vi "Stimulus-Set Level (array).vi"(0 "AO Control in":T1[](array[typedef]) {"Filter"."IIR Filter Cluster"."Forward Coefficients" format="%.4f"; "Filter"."IIR Filter Cluster"."Reverse Coefficients" format="%.4f"}, 1 "Apply multiplier? (F)":bool, 5 "Waveform in":dbl[][](array[numeric]), 11 "error in (no error)":errorcluster) -> (4 "AO Control out":T23(array[cluster]) {"Filter"."IIR Filter Cluster"."Forward Coefficients" format="%.4f"; "Filter"."IIR Filter Cluster"."Reverse Coefficients" format="%.4f"}, 6 "Waveform out":dbl[][](array[numeric]), 8 "Multipliers":dbl[](array[numeric]), 10 "Gains":dbl[](array[numeric]), 14 "Ceilings":dbl[](array[numeric]), 15 "error out":errorcluster)   [LabVIEW 2020]
uses:
  Controls/Waveform XCtl/Waveform Data.ctl
  Controls/Waveform XCtl/Waveform Enum.ctl
  Waveform VIs/Tone VIs/Tone Params.ctl
  Waveform VIs/Pulse Train VIs/Pulse Train Params.ctl
  Waveform VIs/Pulse Train VIs/Pulse Polarity.ctl
  Waveform VIs/Pulse Train VIs/PT-Continuous State.ctl
  Waveform VIs/Noise VIs/Noise Params.ctl
  Waveform VIs/File VIs/StimFile-Params.ctl
  Waveform VIs/FM Sweep VIs/FM Sweep Params.ctl
  Waveform VIs/Chirp Train VIs/Chirp Train.ctl
  Waveform VIs/Chirp Train VIs/Chirp Train Params.ctl
  Waveform VIs/Complex Tone VIs/CT-Params.ctl
  Waveform VIs/Complex Tone VIs/CT-Phase Enum.ctl
  Waveform VIs/Complex Tone VIs/CT-Runtime Data.ctl
  Waveform VIs/Moving Ripple VIs/Moving Ripple.ctl
  Waveform VIs/Moving Ripple VIs/Moving Ripple.Params.ctl
  Waveform VIs/Moving Ripple VIs/Moving Ripple.Data.ctl
  Controls/Filter XCtl/Filter Data.ctl
  Controls/Gate XCtl/Gate Data.ctl
  Controls/Level XCtl/Level Data.ctl
  Controls/Level XCtl/Level Units.ctl
  Controls/Stimulus Channel XCtl/Stimulus Channel Data.ctl
  PXI DAQ VIs/DAQ Engine VIs/AO Gain and Multiplier VIs/PXI Multipliers to AO Gains (1D).vi
  Controls/Waveform XCtl/Waveform XCtl.xctl
  Controls/Filter XCtl/Filter XCtl.xctl
  Controls/Gate XCtl/Gate Control.xctl
  Controls/Level XCtl/Level XCtl.xctl
  Controls/Stimulus Channel XCtl/Stimulus Channel.xctl
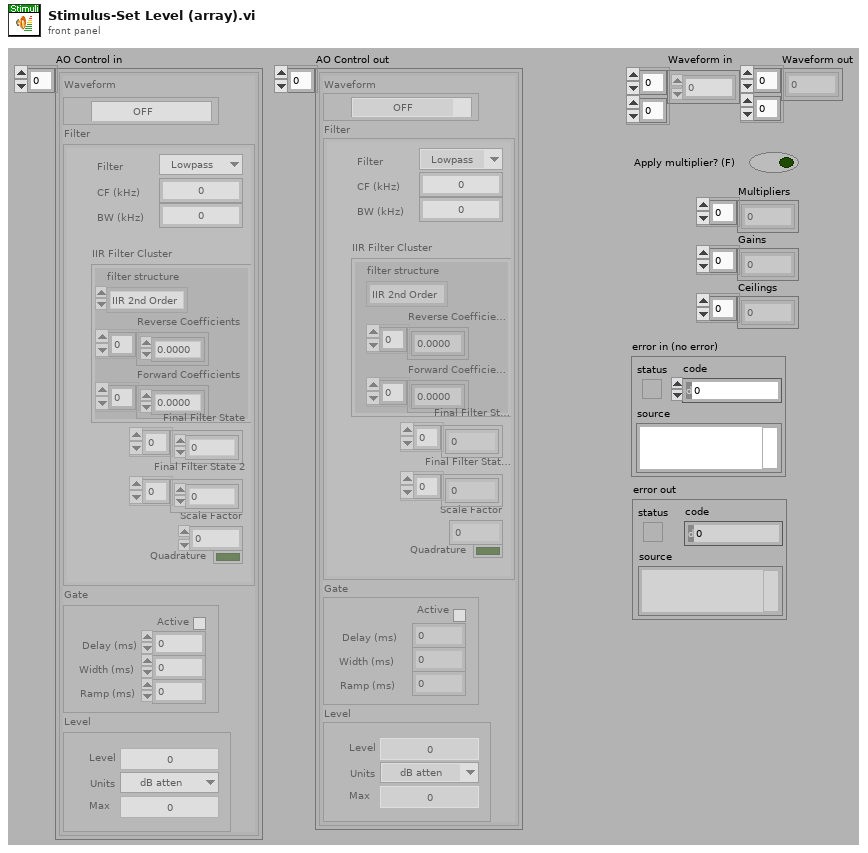
[diagram p1: front panel]
types:
  T1 = typedef "Stimulus Channel.xctl/Stimulus Channel Data.ctl" = cluster{"Waveform":T2, "Filter":T19, "Gate":T20, "Level":T21}
  T2 = typedef "Waveform XCtl.xctl/Waveform Data.ctl" = cluster{"Type":T3, "Tone":T4, "Pulse Train":T5, "Noise":T8, "File":T9, "FMSweep":T10, "Chirp Train":T11, "Complex Tone":cluster{"Params":T13, "Data":T15}, "Moving Ripple":T16}
  T3 = typedef "Waveform Enum.ctl" = enum16{"OFF", "Tone", "Noise", "Pulse Train", "File", "FM Sweep", "Chirp Train", "Complex Tone", "FM Tone", "Moving Ripple"}
  T4 = typedef "Tone Params.ctl" = cluster{"Frequency (kHz)":dbl, "Last Freq":dbl, "Last Phase":dbl}
  T5 = typedef "Pulse Train Params.ctl" = cluster{"Pulse width (us)":dbl, "Pulse rate (Hz)":dbl, "Gap (ms)":dbl, "Polarity":T6, "PT State":T7, "Asynch":bool}
  T6 = typedef "Pulse Polarity.ctl" = enum16{"POS", "NEG", "POS-NEG", "NEG-POS"}
  T7 = typedef "PT-Continuous State.ctl" = cluster{"Template":dbl[], "Nperiod":i32, "Index":i32, "Pulse Rate (Hz)":dbl, "Phase (cycles)":dbl, "Noff":i32}
  T8 = typedef "Noise Params.ctl" = cluster{"InvFilt":bool, "Noise":dbl[], "CurPt":i32, "Aweight":bool, "Seed":i32, "afile":path}
  T9 = typedef "StimFile-Params.ctl" = cluster{"Filename":path, "Signal":dbl[], "Channel":i32, "stream":bool, "offset":i32, "nreps":i32, "loops":i32, "Randomize":bool, "order":i32[], "Seed":i32, "Tokens":i32}
  T10 = typedef "FM Sweep Params.ctl" = cluster{"Rate (oct/s)":dbl, "Fmin (Hz)":dbl, "Fmax (Hz)":dbl, "Ramp (ms)":dbl, "Linear":bool}
  T11 = typedef "Chirp Train.ctl" = cluster{"Params":T12, "Data":cluster{"WF":dbl[]}}
  T12 = typedef "Chirp Train Params.ctl" = cluster{"Fmin (kHz)":dbl, "Fmax (kHz)":dbl, "Compensate":bool, "Duration (ms)":dbl}
  T13 = typedef "CT-Params.ctl" = cluster{"F0 (Hz)":dbl, "Band":cluster{"Flow (Hz)":dbl, "Fhigh (Hz)":dbl}, "Phase":T14, "Min F0 (Hz)":dbl, "Max F0 (Hz)":dbl, "ContinRandPhase":bool, "Max peak factor":dbl, "Max mod depth":dbl, "MinHarmNum":i32, "MaxHarmNum":i32, "Level Mode":enum16{"per component", "overall rms"}, "% jitter":dbl}
  T14 = typedef "CT-Phase Enum.ctl" = enum16{"Cosine", "Random", "Alternating"}
  T15 = typedef "CT-Runtime Data.ctl" = cluster{"Ncomp":i32, "MinHarm":i32, "Phase":dbl[], "Amplitude":dbl[], "Npts/frame":i32, "Last F0":dbl, "Fmin":dbl, "Fmax":dbl, "Lslope":dbl, "randphase":bool, "overall rms":bool, "fmult":dbl[], "jittered":bool}
  T16 = typedef "Moving Ripple.ctl" = cluster{"Params":T17, "Data":T18}
  T17 = typedef "Moving Ripple.Params.ctl" = cluster{"Fmin":dbl, "Fmax":dbl, "Density":dbl, "Velocity":dbl, "Depth":dbl, "Phase":dbl, "Comp/oct":i32}
  T18 = typedef "Moving Ripple.Data.ctl" = cluster{"Freq":dbl[], "A":dbl[], "phase":dbl[], "Phase":dbl}
  T19 = typedef "Filter XCtl.xctl/Filter Data.ctl" = cluster{"CF (kHz)":dbl, "BW (kHz)":dbl, "IIR Filter Cluster":cluster{"filter structure":enum32{"IIR 2nd Order", "IIR 4th Order"}, "Reverse Coefficients":dbl[], "Forward Coefficients":dbl[]}, "Final Filter State":dbl[], "Scale Factor":dbl, "Final Filter State 2":dbl[], "Quadrature":bool, "Type":enum16{"Lowpass", "Highpass", "Bandpass", "Bandstop", "OFF"}}
  T20 = typedef "Gate Control.xctl/Gate Data.ctl" = cluster{"Active":bool, "Delay (ms)":dbl, "Width (ms)":dbl, "Ramp (ms)":dbl}
  T21 = typedef "Level XCtl.xctl/Level Data.ctl" = cluster{"Level":dbl, "Units":T22, "Max":dbl, "Multiplier":dbl, "Cal File":path, "Cal":cluster{"Freq (Hz)":dbl[], "Mag (dB SPL)":dbl[], "Phase (deg)":dbl[]}}
  T22 = typedef "Level Units.ctl" = enum16{"dB atten", "dB SPL", "dB re 1 Vrms", "dB V/Hz½", "mW", "dB HL", "Volts", "dB mW"}
  T23 = cluster{"Waveform":T2, "Filter":T19, "Gate":T20, "Level":T21}[]
  T24 = cluster{"Waveform":T2, "Filter":T19, "Gate":T20, "Level":T21}
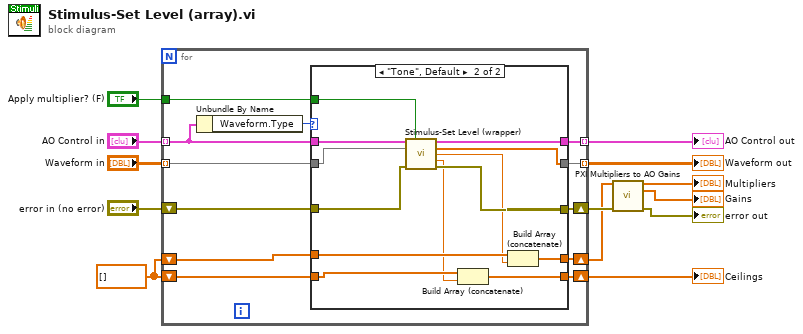
[diagram p0: block diagram]
diagram:
  w7 = dbl[] []
  n1 = for {
    tunnel: [w23] -> w2 mode=indexing
    shift-right: [w21] -> w8
    shift-left: w7 -> [w22]
    shift-right: [w24] -> w12
    shift-left: "error in (no error)" -> [w25]
    shift-right: [w19] -> w6
    shift-left: w7 -> [w20]
    tunnel: "AO Control in" -> [w14] mode=indexing
    tunnel: "Waveform in" -> [w17] mode=indexing
    tunnel: [w16] -> w4 mode=indexing
    tunnel: "Apply multiplier? (F)" -> [w15]
    n2 = Unbundle By Name(w14) -> ("Waveform.Type"=w18:T3)
    n3 = case shown="\"Tone\", Default" w18 {
      tunnel: w25 -> [w30 w34]
      tunnel: [w30 w39] -> w24
      tunnel: [w27 w38] -> w23
      tunnel: w22 -> [w29 w42]
      tunnel: [w29 w43] -> w21
      tunnel: w20 -> [w28 w40]
      tunnel: [w28 w41] -> w19
      tunnel: w14 -> [w27 w35]
      tunnel: w17 -> [w26 w33]
      tunnel: [w26 w32] -> w16
      tunnel: w15 -> [_ w31]
      frame "OFF" {
      }
      frame "Tone", Default {
        n4 = call "Stimulus-Set Level (wrapper).vi"("Stimulus Channel"=w35, "Apply multiplier? (F)"=w31, "Waveform in"=w33, "error in (no error)"=w34) -> ("Stimulus Channel out"=w38:T24, "Waveform out"=w32:dbl[], "Multiplier"=w36:dbl, "Ceiling"=w37:dbl, "error out"=w39:errorcluster)  [unwired: 7 in]
        n5 = Build Array (concatenate)(w40, w37) -> (w41:dbl[])
        n6 = Build Array (concatenate)(w42, w36) -> (w43:dbl[])
      }
    }
  }
  "Ceilings" <- w6
  "Waveform out" <- w4
  "AO Control out" <- w2
  n7 = call-poly "PXI Multipliers to AO Gains.vi"("Multipliers in"=w8, "error in (no error)"=w12) -> ("Multipliers out"=→"Multipliers":dbl[], "Gains"=→"Gains":dbl[], "error out"=→"error out":errorcluster)  [unwired: 11 in]
